vi "_blacklist.vi"() -> (3 "blacklist":string[](array[string]))   [LabVIEW 2017, in "TagDB RefManager.lvlib"]
uses:
  TagDB RefManager.lvlib
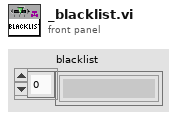
[diagram p1: front panel]
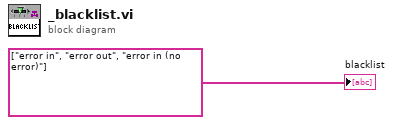
[diagram p0: block diagram]
diagram:
  "blacklist" <- string[] ["error in", "error out", "error in (no error)"] ("blacklist")
